vi "Read Voltaje.vi"(8 "error in (no error)":errorcluster, 11 "Fuente de poder in":refnum<class "Fuente de poder.lvclass">) -> (0 "error out":errorcluster, 2 "Voltaje":dbl, 3 "Fuente de poder out":refnum<class "Fuente de poder.lvclass">)   [LabVIEW 2020, in "Fuente de poder.lvclass"]
uses:
  Fuente de poder.lvclass
  Fuente de poder.lvclass/Fuente de poder.ctl
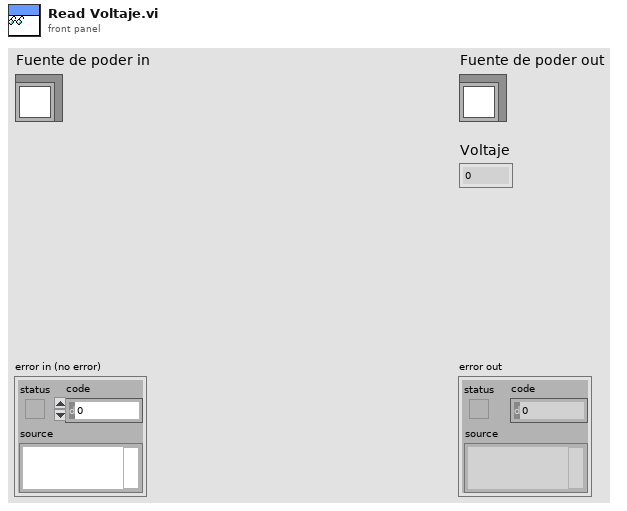
[diagram p1: front panel]
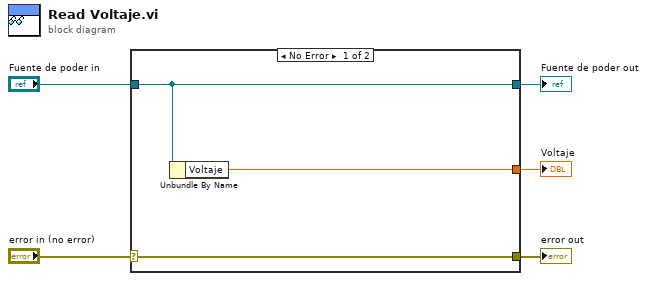
[diagram p0: block diagram]
diagram:
  n1 = case shown="No Error" "error in (no error)" {
    selector: "error in (no error)" -> [w8 w9]
    tunnel: [w8 w9] -> w4
    tunnel: [w7 w10] -> w2
    tunnel: "Fuente de poder in" -> [w7 w10]
    tunnel: [w6 _] -> w1
    frame No Error {
      n2 = Unbundle By Name(w7) -> ("Voltaje"=w6:dbl)
    }
    frame Error {
    }
  }
  "error out" <- w4
  "Fuente de poder out" <- w2
  "Voltaje" <- w1
